vi "mcc_etc_read.vi"(8 "error in":errorcluster, 11 "task in":refnum<k24>) -> (0 "error out":errorcluster={"status"=TRUE, "code"=10023, "source"="ULx Create Channel (AI-Voltage-Basic).vi:5780001<ERR>\nMeasurements: Channel not specified."}, 1 "status":bool=TRUE, 2 "temperature_array":dbl[](array[numeric]), 3 "task out":refnum<k24>)   [LabVIEW 2019]
uses:
  C:/Program Files/National Instruments/LabVIEW 2019/vi.lib/ULx/ULx_LV.dll
  Program Files/National Instruments/LabVIEW 2019/vi.lib/ULx/ULx_LV.dll
  <vilib>/ULx/Read.llb/ULx Read (Analog 1D DBL NChan 1Samp).vi
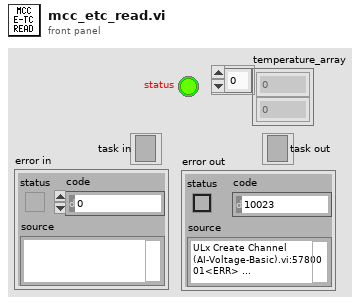
[diagram p1: front panel]
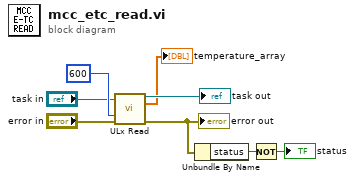
[diagram p0: block diagram]
diagram:
  n1 = call-poly <vilib>:"ULx Read.vi"("task in"="task in", "timeout"=600, "error in"="error in") -> ("task out"=→"task out":refnum<k24>, "data"=→"temperature_array":dbl[], "error out"=w4:errorcluster)  [unwired: 10 in]
  "error out" <- w4
  n2 = Unbundle By Name(w4) -> ("status"=w3:bool)
  n3 = Not(x=w3) -> (.not. x?=→"status":bool)
